vi "WriteMotorInfoToMap.vi"(8 "error in (no error)":errorcluster, 10 "Map in":T7, 11 "Group":T1) -> (0 "error out":errorcluster, 2 "Map out":T7, 3 "Group out":T1)   [LabVIEW 2017, in "McsaAnalysisHighRate.lvlib"]
uses:
  <vilib>/addons/InsightCM/Devices/Shared/Mcsa/McsaAnalysisHighRate/McsaAnalysisHighRate.lvlib
  <vilib>/addons/PointValueMap/controls/PointMap.ctl
  <vilib>/addons/InsightCM/Devices/Shared/Mcsa/McsaAnalysisHighRate/controls/Group.ctl
  <vilib>/addons/InsightCM/Utilities/Analysis/MCSA/controls/McsaChannel.ctl
  <vilib>/addons/InsightCM/Utilities/Analysis/Shared/controls/Feature.ctl
  <vilib>/addons/InsightCM/Utilities/Analysis/Shared/controls/AmplitudeScale.ctl
  <vilib>/addons/InsightCM/MessageBus/Base/controls/KeyValuePair.ctl
  <vilib>/addons/InsightCM/Utilities/Analysis/MCSA/controls/McsaMotor.ctl
  <vilib>/addons/InsightCM/Utilities/MCSA/McsaUtilities.lvlib
  <vilib>/addons/PointValueMap/PointValueMap.lvlib
  <vilib>/addons/InsightCM/Utilities/Analysis/Shared/AnalysisHelper.lvlib
  <vilib>/addons/InsightCM/Utilities/Analysis/MCSA/McsaAnalysisFunctions.lvlib
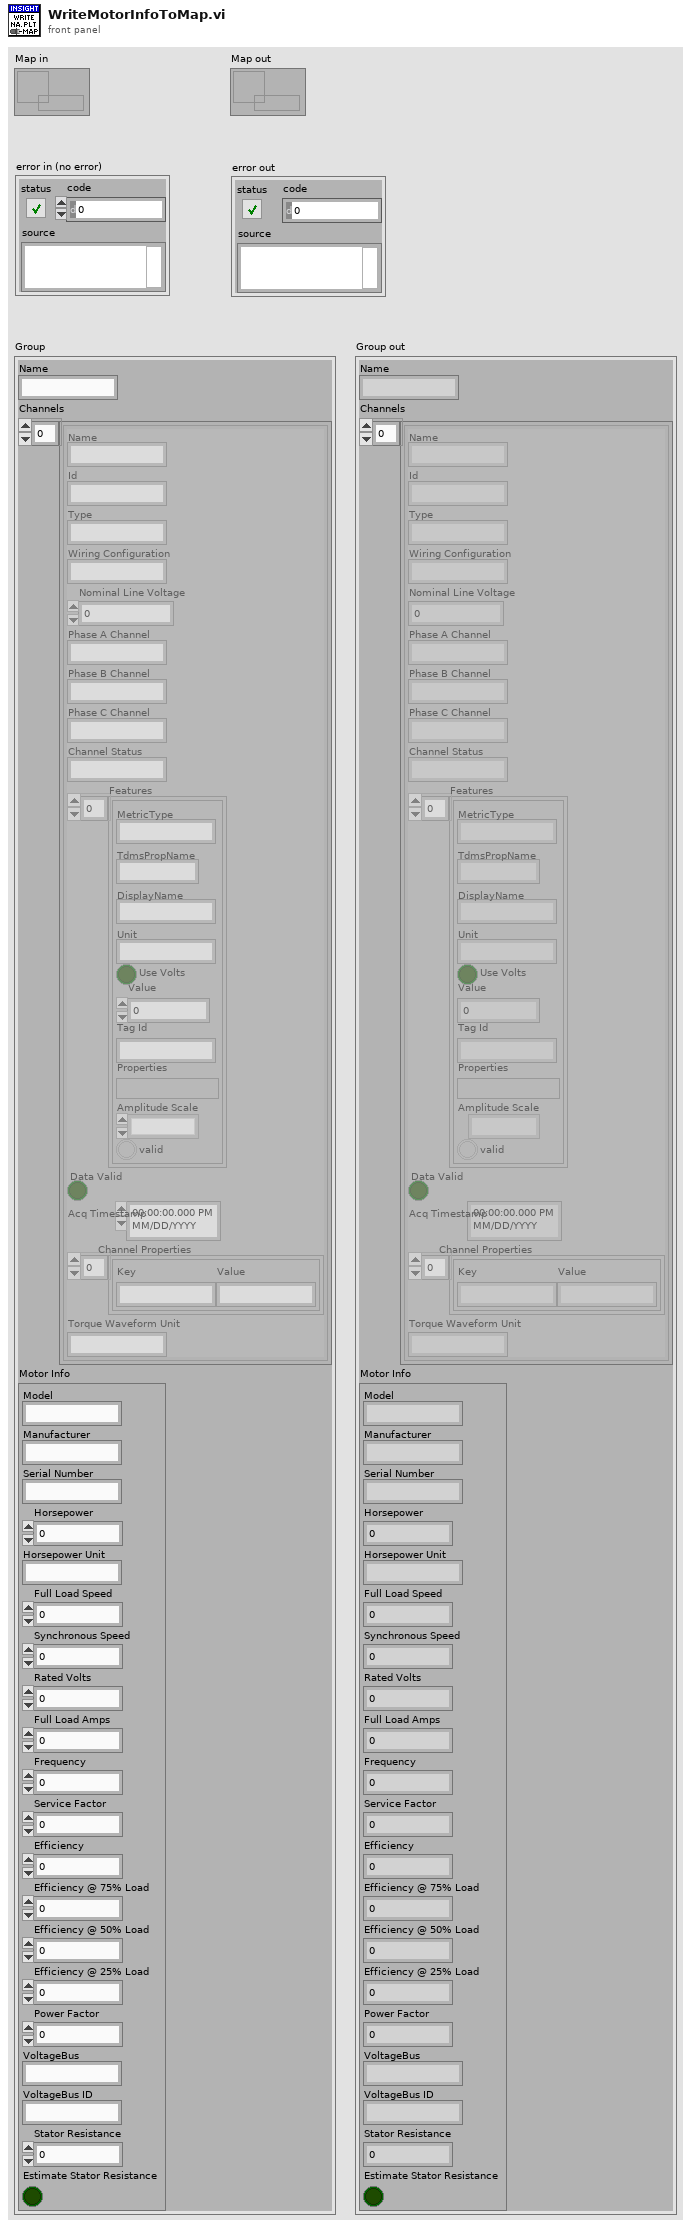
[diagram p1: front panel]
types:
  T1 = typedef "McsaAnalysisHighRate.lvlib/Group.ctl" = cluster{"Name":string, "Channels":T2[], "Motor Info":T6}
  T2 = typedef "McsaAnalysisFunctions.lvlib/McsaChannel.ctl" = cluster{"Name":string, "Id":string, "Type":string, "Wiring Configuration":string, "Nominal Line Voltage":dbl, "Phase A Channel":string, "Phase B Channel":string, "Phase C Channel":string, "Channel Status":string, "Features":T3[], "Data Valid":bool, "Acq Timestamp":timestamp, "Channel Properties":T5[], "Torque Waveform Unit":string}
  T3 = typedef "AnalysisHelper.lvlib/Feature.ctl" = cluster{"MetricType":string, "TdmsPropName":string, "DisplayName":string, "Unit":string, "Use Volts":bool, "Value":dbl, "Tag Id":string, "Properties":variant, "Amplitude Scale":T4, "valid":bool}
  T4 = typedef "AnalysisHelper.lvlib/AmplitudeScale.ctl" = enum16{"rms", "peak", "pk-pk"}
  T5 = typedef "KeyValuePair.ctl" = cluster{"Key":string, "Value":string}
  T6 = typedef "McsaAnalysisFunctions.lvlib/McsaMotor.ctl" = cluster{"Model":string, "Manufacturer":string, "Serial Number":string, "Horsepower":dbl, "Horsepower Unit":string, "Full Load Speed":dbl, "Synchronous Speed":dbl, "Rated Volts":dbl, "Full Load Amps":dbl, "Frequency":dbl, "Service Factor":dbl, "Efficiency":dbl, "Efficiency @ 75% Load":dbl, "Efficiency @ 50% Load":dbl, "Efficiency @ 25% Load":dbl, "Power Factor":dbl, "VoltageBus":string, "VoltageBus ID":string, "Stator Resistance":dbl, "Estimate Stator Resistance":bool}
  T7 = typedef "PointValueMap.lvlib/PointMap.ctl" = refnum<data-value>
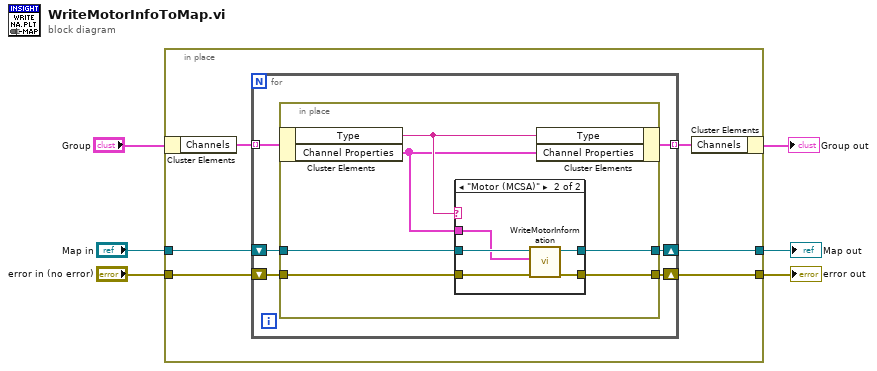
[diagram p0: block diagram]
diagram:
  n1 = in-place {
    in-place-border: "Map in" -> [w8]
    in-place-border: "error in (no error)" -> [w12]
    in-place-border: [w10] -> w2
    in-place-border: [w7] -> w1
    n2 = in-place-cluster #1("Group") -> ("Channels"=w11:T2[])
    n3 = for {
      tunnel: w11 -> [w16] mode=indexing
      tunnel: [w15] -> w9 mode=indexing
      shift-right: [w17] -> w10
      shift-left: w12 -> [w18]
      shift-right: [w13] -> w7
      shift-left: w8 -> [w14]
      n4 = in-place {
        in-place-border: w18 -> [w24]
        in-place-border: [w23] -> w17
        in-place-border: w14 -> [w20]
        in-place-border: [w19] -> w13
        n5 = in-place-cluster #2(w16) -> ("Type"=w22:string, "Channel Properties"=w21:T5[])
        n6 = case shown="\"Motor (MCSA)\"" w22 {
          tunnel: w24 -> [w25 w31]
          tunnel: [w25 w29] -> w23
          tunnel: w21 -> [_ w27]
          tunnel: w20 -> [w26 w30]
          tunnel: [w26 w28] -> w19
          frame Default {
          }
          frame "Motor (MCSA)" {
            n7 = call <vilib>:"WriteMotorInformation.vi"("error in (no error)"=w31, "Properties"=w27, "map in"=w30) -> ("error out"=w29:errorcluster, "map out"=w28:T7)  [unwired: 7 in]
          }
        }
        n8 = in-place-cluster #2("Type"=w22, "Channel Properties"=w21) -> (w15:T2)
      }
    }
    n9 = in-place-cluster #1("Channels"=w9) -> (→"Group out":T1)
  }
  "error out" <- w2
  "Map out" <- w1
